vi "hermes lead to destination manager.vi"   [LabVIEW 2010, in "Test.lvrbt"]
uses:
  Test.lvrbt
  <vilib>/NXT/Dual Mode Library/Display/clearDisplay.vi
  <vilib>/NXT/Dual Mode Library/Display/drawText.vi
  <vilib>/NXT/Dual Mode Library/prims/maxAndMin/maxAndMin_int.vi
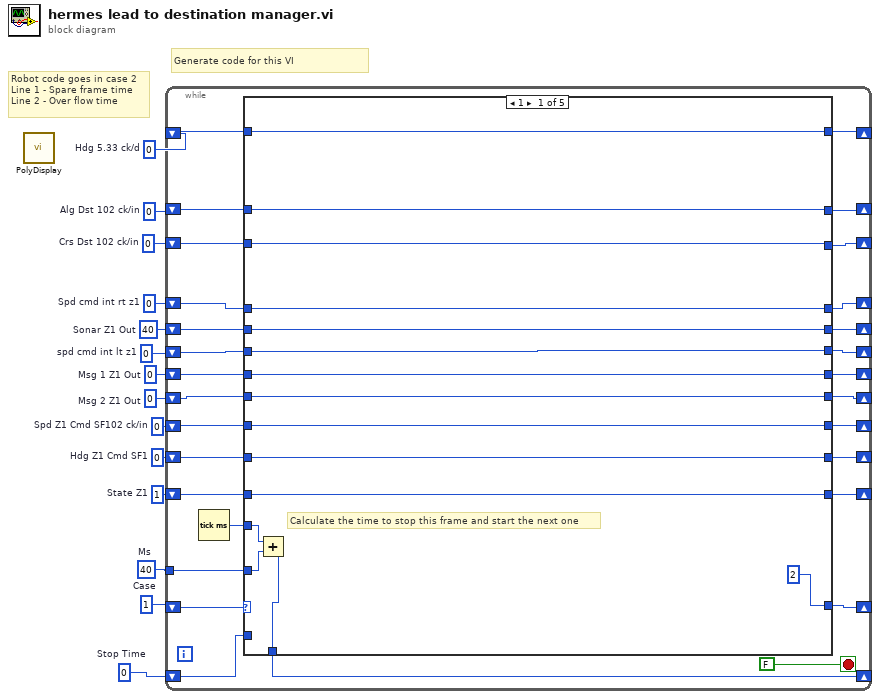
[diagram p0: block diagram]
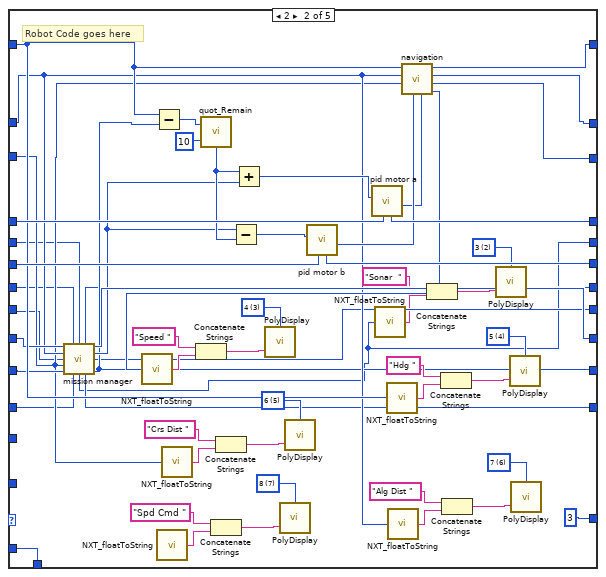
[diagram p2: hidden frame]
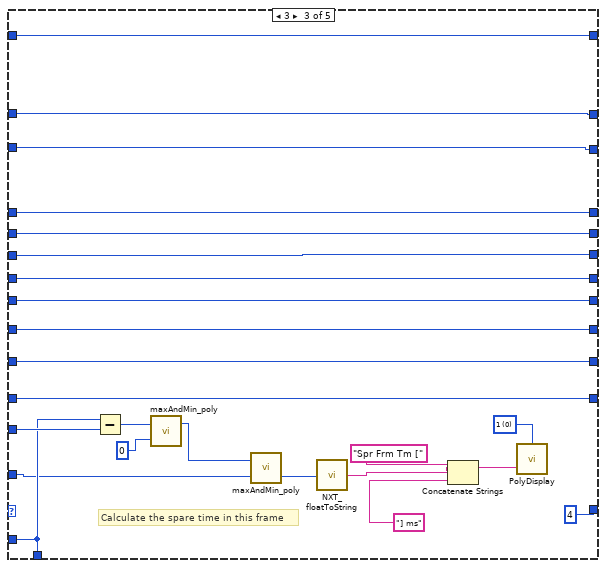
[diagram p3: hidden frame]
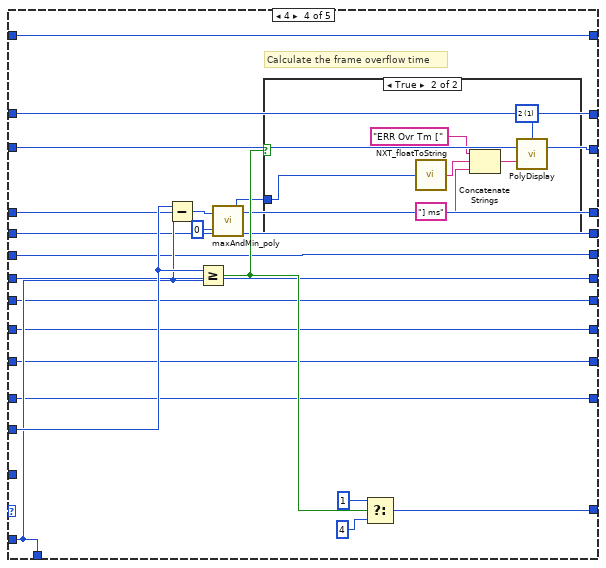
[diagram p4: hidden frame]
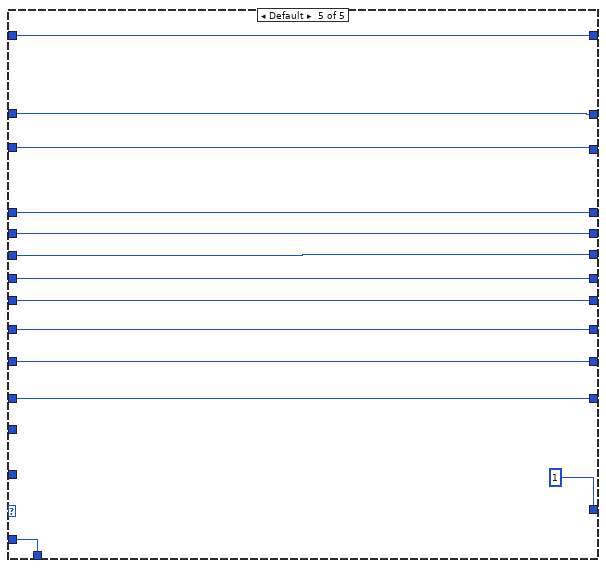
[diagram p6: hidden frame]
diagram:
  w1 = i16 40  # Sonar Z1 Out
  w2 = 0  # Msg 2 Z1 Out
  w3 = 0  # Msg 1 Z1 Out
  w4 = 0  # Spd Z1 Cmd SF102 ck/in
  w5 = 0  # Hdg Z1 Cmd SF1
  w6 = 1  # State Z1
  w7 = 0  # Crs Dst 102 ck/in
  w8 = 0  # Hdg 5.33 ck/d
  w9 = 0  # Alg Dst 102 ck/in
  w10 = 0  # spd cmd int lt z1
  w11 = 0  # Spd cmd int rt z1
  w12 = u32 40  # Ms
  w13 = u32 0  # Stop Time
  w14 = 1  # Case
  # "Generate code for this VI"
  # "Robot code goes in case 2\nLine 1 - Spare frame time\nLine 2 - Over flow time"
  n1 = call-poly <vilib>:"PolyDisplay.vi"() -> ()  [unwired: 4 in, 1 out]
  n2 = while {
    shift-right: [w42] -> _
    shift-left: w14 -> [w43]
    shift-right: [w38] -> _
    shift-left: w13 -> [w40]
    tunnel: w12 -> [w39]
    shift-right: [w36] -> _
    shift-left: w11 -> [w35]
    shift-right: [w33] -> _
    shift-left: w10 -> [w34]
    shift-right: [w32] -> _
    shift-left: w8 -> [w30]
    shift-right: [w31] -> _
    shift-left: w9 -> [w29]
    shift-right: [w27] -> _
    shift-left: w7 -> [w28]
    shift-right: [w25] -> _
    shift-left: w4 -> [w26]
    shift-right: [w23] -> _
    shift-left: w5 -> [w24]
    shift-right: [w21] -> _
    shift-left: w6 -> [w22]
    shift-right: [w20] -> _
    shift-left: w3 -> [w19]
    shift-right: [w17] -> _
    shift-left: w2 -> [w18]
    shift-right: [w16] -> _
    shift-left: w1 -> [w15]
    stop <- FALSE stop-if-true
    n3 = Tick Count (ms)() -> (millisecond timer value=w41:u32)
    n4 = case shown="1" w43 {
      tunnel: [2 3 4 w157 1 ("t")] -> w42
      tunnel: w41 -> [w57 _ w133 w156 _]
      tunnel: w40 -> [_ w115 w132 w155 w177]
      tunnel: w39 -> [w56 _ w129 _ _]
      tunnel: [w55 w115 w132 w155 w177] -> w38
      tunnel: [w54 w109 w126 w150 w176] -> w36
      tunnel: w35 -> [w54 w108 w126 w150 w176]
      tunnel: w34 -> [w53 w106 w125 w149 w175]
      tunnel: [w53 w107 w125 w149 w175] -> w33
      tunnel: [w51 w101 w123 w147 w173] -> w32
      tunnel: [w52 w105 w124 w148 w174] -> w31
      tunnel: w30 -> [w51 w91 w123 w147 w173]
      tunnel: w29 -> [w52 w73 w124 w148 w174]
      tunnel: w28 -> [w50 w72 w122 w146 w172]
      tunnel: [w50 w102 w122 w146 w172] -> w27
      tunnel: w26 -> [w49 w77 w121 w143 w169]
      tunnel: [w49 w76 w121 w143 w169] -> w25
      tunnel: w24 -> [w48 w75 w120 w144 w170]
      tunnel: [w48 w71 w120 w144 w170] -> w23
      tunnel: w22 -> [w47 w63 w119 w145 w171]
      tunnel: [w47 w62 w119 w145 w171] -> w21
      tunnel: [w46 w70 w118 w141 w167] -> w20
      tunnel: w19 -> [w46 w69 w118 w141 w167]
      tunnel: w18 -> [w45 w61 w117 w142 w168]
      tunnel: [w45 w68 w117 w142 w168] -> w17
      tunnel: [w44 w60 w116 w140 w166] -> w16
      tunnel: w15 -> [w44 w59 w116 w140 w166]
      frame 1 {
        # "Calculate the time to stop this frame and start the next one"
        n5 = Add(x=w57, y=w56) -> (x+y=w55:u32)
      }
      frame 2 {
        w67 = i16 2 items=["1", "2", "3", "4", "5", "6", "7", "8"] ("Line")
        w81 = i16 7 items=["1", "2", "3", "4", "5", "6", "7", "8"] ("Line")
        w85 = i16 5 items=["1", "2", "3", "4", "5", "6", "7", "8"] ("Line")
        w89 = i16 6 items=["1", "2", "3", "4", "5", "6", "7", "8"] ("Line")
        w96 = i16 3 items=["1", "2", "3", "4", "5", "6", "7", "8"] ("Line")
        w113 = i16 4 items=["1", "2", "3", "4", "5", "6", "7", "8"] ("Line")
        # "Robot Code goes here"
        n6 = call "mission manager.vi"("Spd Z1 In Cmd"=w77, "Msg 1 Z1 In"=w69, "Sonar Z1 In"=w59, "Alg In SF102 ck/in"=w73, "Msg 2 Z1 In"=w61, "Cros In SF102 ck/in"=w72, "Hdg Z1 In Cmd"=w75, "State Z1 In"=w63) -> ("Msg 1 Z1 Out"=w70:i32, "Spd Z1 Out Cmd 32.64 ck s/in cy"=w76:i32, "Spd Out Cmd SF SF4.08 ck s/in cy"=w74:i32, "Msg 2 Z1 Out"=w68:i32, "Sonar Z1 Out"=w60:i16, "State Z1 Out"=w62:i8, "Hdg Z1 Out Cmd SF 5.33 ck/dg"=w71:i32)  [unwired: 1 in]
        n7 = Subtract(x=w91, y=w71) -> (x-y=w90:i32)
        n8 = call <vilib>:"NXT_floatToString.vi"() -> ("string"=w79:string)  [unwired: 1 in]
        n9 = call <vilib>:"NXT_floatToString.vi"("number"=w72) -> ("string"=w83:string)
        n10 = call <vilib>:"quot_Remain.vi"("y"=10, "x"=w90) -> ("floor(x/y)"=w100:i32)  [unwired: 1 out]
        n11 = Concatenate Strings("Spd Cmd " ("Text"), w79) -> (w78:string)
        n12 = Concatenate Strings("Crs Dist " ("Text"), w83) -> (w82:string)
        n13 = Subtract(x=w74, y=w100) -> (x-y=w97:i32)
        n14 = Add(x=w100, y=w74) -> (x+y=w98:i32)
        n15 = call-poly <vilib>:"PolyDisplay.vi"("Text"=w78, "Line"=w81) -> ()  [unwired: 2 in, 1 out]
        n16 = call-poly <vilib>:"PolyDisplay.vi"("Text"=w82, "Line"=w85) -> ()  [unwired: 2 in, 1 out]
        n17 = call "pid motor b.vi"("Int Z1 In"=w106, "Spd Cmd"=w97) -> ("Motor Speed"=w104:i32, "Int Z1 Out"=w107:i32)  [unwired: 6 in, 2 out]
        n18 = call "pid motor a.vi"("Int Z1 In"=w108, "Spd Cmd SF51 ck/in"=w98) -> ("Spd SF 51 ck/in"=w103:i32, "Int Z1 Out"=w109:i32)  [unwired: 6 in, 2 out]
        n19 = call <vilib>:"NXT_floatToString.vi"("number"=w60) -> ("string"=w65:string)
        n20 = call <vilib>:"NXT_floatToString.vi"("number"=w91) -> ("string"=w111:string)
        n21 = call <vilib>:"NXT_floatToString.vi"("number"=w73) -> ("string"=w87:string)
        n22 = call "navigation.vi"("Right Motor Speed"=w103, "Left Motor Speed"=w104, "Cross Dist Z1 In"=w72, "Along Dist Z1 In"=w73, "Hdg Z1 In"=w91) -> ("Speed"=w92:i32, "Cross Dist Z1 Out SF102 ck/in"=w102:i32, "Along Dist Z1 Out SF102 ck/in"=w105:i32, "Hdg Z1 Out SF 5.33 ck/dg"=w101:i32)  [unwired: 3 in]
        n23 = call <vilib>:"NXT_floatToString.vi"("number"=w92) -> ("string"=w94:string)
        n24 = Concatenate Strings("Speed " ("Text"), w94) -> (w93:string)
        n25 = call-poly <vilib>:"PolyDisplay.vi"("Text"=w93, "Line"=w96) -> ()  [unwired: 2 in, 1 out]
        n26 = Concatenate Strings("Sonar  " ("Text"), w65) -> (w64:string)
        n27 = Concatenate Strings("Hdg " ("Text"), w111) -> (w110:string)
        n28 = Concatenate Strings("Alg Dist " ("Text"), w87) -> (w86:string)
        n29 = call-poly <vilib>:"PolyDisplay.vi"("Text"=w64, "Line"=w67) -> ()  [unwired: 2 in, 1 out]
        n30 = call-poly <vilib>:"PolyDisplay.vi"("Text"=w110, "Line"=w113) -> ()  [unwired: 2 in, 1 out]
        n31 = call-poly <vilib>:"PolyDisplay.vi"("Text"=w86, "Line"=w89) -> ()  [unwired: 2 in, 1 out]
      }
      frame 3 {
        w138 = i16 0 items=["1", "2", "3", "4", "5", "6", "7", "8"] ("Line")
        # "Calculate the spare time in this frame"
        n32 = Subtract(x=w132, y=w133) -> (x-y=w130:u32)
        n33 = call-poly <vilib>:"maxAndMin_poly.vi"("y"=0, "x"=w130) -> ("max(x,y)"=w128:i32)  [unwired: 1 out]
        n34 = call-poly <vilib>:"maxAndMin_poly.vi"("y"=w129, "x"=w128) -> ("min(x,y)"=w127:i32)  [unwired: 1 out]
        n35 = call <vilib>:"NXT_floatToString.vi"("number"=w127) -> ("string"=w136:string)
        n36 = Concatenate Strings("Spr Frm Tm [" ("Text"), w136, "] ms" ("string")) -> (w135:string)
        n37 = call-poly <vilib>:"PolyDisplay.vi"("Text"=w135, "Line"=w138) -> ()  [unwired: 2 in, 1 out]
      }
      frame 4 {
        # "Calculate the frame overflow time"
        n38 = Subtract(x=w156, y=w155) -> (x-y=w153:u32)
        n39 = Greater Or Equal?(x=w156, y=w155) -> (x >= y?=w154:bool)
        n40 = call-poly <vilib>:"maxAndMin_poly.vi"("y"=0, "x"=w153) -> ("max(x,y)"=w151:i32)  [unwired: 1 out]
        n41 = case shown="True" w154 {
          tunnel: w151 -> [_ w160]
          frame False {
          }
          frame True {
            w165 = i16 1 items=["1", "2", "3", "4", "5", "6", "7", "8"] ("Line")
            n42 = call <vilib>:"NXT_floatToString.vi"("number"=w160) -> ("string"=w164:string)
            n43 = Concatenate Strings("ERR Ovr Tm [" ("Text"), w164, "] ms" ("string")) -> (w163:string)
            n44 = call-poly <vilib>:"PolyDisplay.vi"("Text"=w163, "Line"=w165) -> ()  [unwired: 2 in, 1 out]
          }
        }
        n45 = Select(t=1, s=w154, f=4) -> (s? t:f=w157:i32)
      }
      frame Default {
      }
    }
  }
